vi "getTaskChannel.vi"(8 "error in (no error)":errorcluster, 11 "ITask in":refnum<class "ITask.lvclass">) -> (0 "error out":errorcluster, 2 "taskChannel":refnum<class "ITaskChannel.lvclass">, 3 "ITask out":refnum<class "ITask.lvclass">)   [LabVIEW 2023, in "TLC_Daemon.lvlib" / "ITask.lvclass"]
doc: "Returns the Task Channel type used by the task."
uses:
  ITask.lvclass
  ITaskChannel/ITaskChannel.lvclass
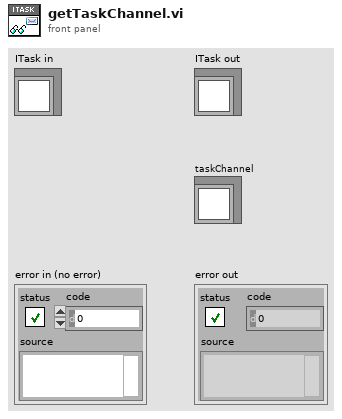
[diagram p1: front panel]
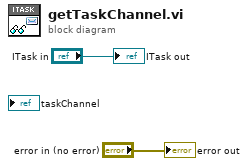
[diagram p0: block diagram]
diagram:
  "error out" <- "error in (no error)"
  "ITask out" <- "ITask in"
